vi "BUILD_uninstall core.vi"(6 "Buildlog":path, 8 "error in":errorcluster, 9 "args":string[](array[string]), 11 "appended path":path) -> (0 "error out":errorcluster)   [LabVIEW 2010]
uses:
  <vilib>/JKI/VIPM API/VIPM API_vipm_api.lvlib
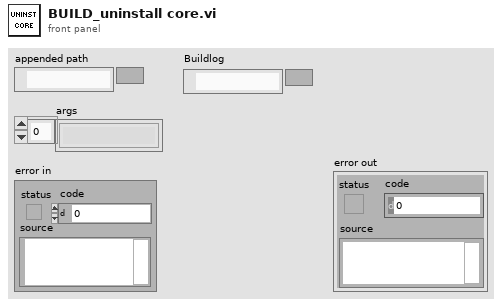
[diagram p1: front panel]
types:
  T1 = typedef "VIPM API_vipm_api.lvlib/Library Contents Cluster_vipm_api.ctl" = cluster{"Package Name":string, "Version":string, "Display Name":string, "Repository Name":string, "Company Name":string, "License Type":string, "Installed":bool, "Deprecated":bool, "Dependency or Conflict Problem":bool, "Downloaded":bool}
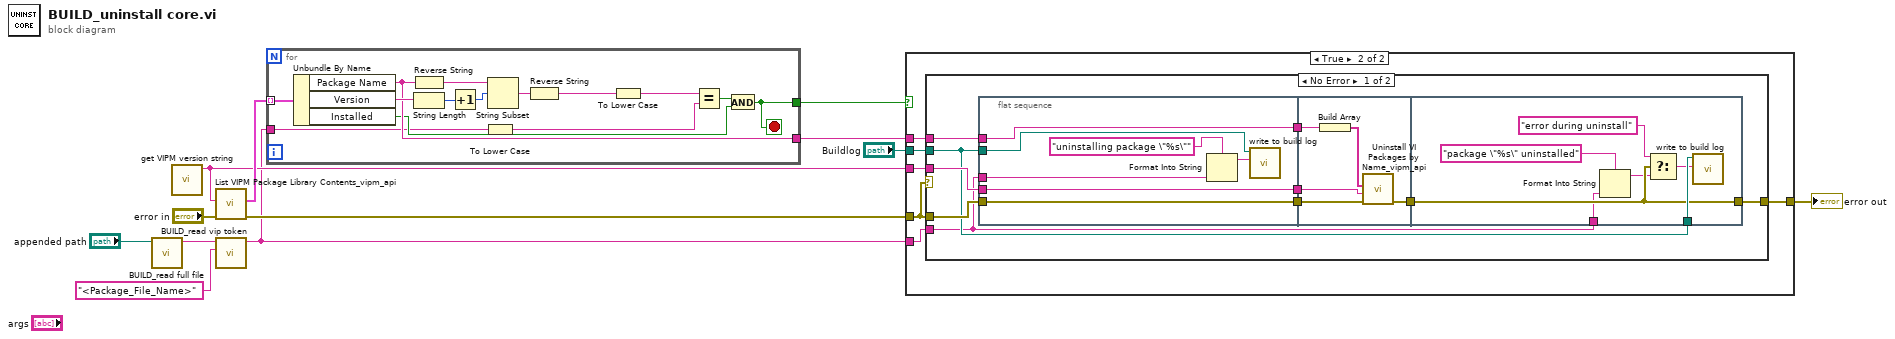
[diagram p0: block diagram]
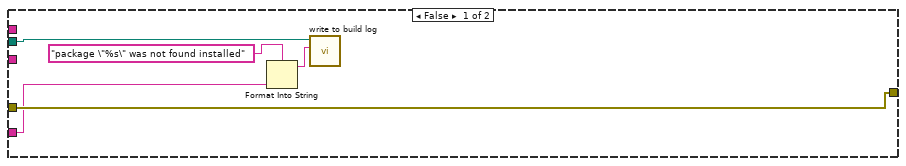
[diagram p2: hidden frame]
diagram:
  n1 = call "BUILD_read full file.vi"("vip file"="appended path") -> ("data"=w11:string)  [unwired: 9 in, 1 out]
  n2 = call "get VIPM version string.vi"() -> ("version string"=w3:string)  [unwired: 11 in]
  n3 = call <vilib>:"List VIPM Package Library Contents_vipm_api.vi"("error in (no error)"="error in", "LabVIEW Version"=w3) -> ("error out"=w7:errorcluster, "Library Contents []"=w6:T1[])  [unwired: 8 in]
  n4 = call "BUILD_read vip token.vi"("regular expression"="<Package_File_Name>", "data"=w11) -> ("trimmed string"=w1:string)  [unwired: 8 in, 1 out]
  n5 = for {
    tunnel: w6 -> [w26] mode=indexing
    tunnel: [w20] -> w8
    tunnel: [w16] -> w9
    tunnel: w1 -> [w15]
    stop <- w16 stop-if-true
    n6 = Unbundle By Name(w26) -> ("Package Name"=w20:string, "Version"=w25:string, "Installed"=w17:bool)
    n7 = Reverse String(1:w20) -> (0:w22:string)
    n8 = String Length(string=w25) -> (length=w24:i32)
    n9 = Increment(x=w24) -> (x+1=w23:i32)
    n10 = To Lower Case(string=w15) -> (all lower case string=w13:string)
    n11 = String Subset(string=w22, offset (0)=w23) -> (substring=w21:string)  [unwired: 1 in]
    n12 = Reverse String(1:w21) -> (0:w19:string)
    n13 = To Lower Case(string=w19) -> (all lower case string=w14:string)
    n14 = Equal?(x=w14, y=w13) -> (x = y?=w18:bool)
    n15 = And(x=w18, y=w17) -> (x .and. y?=w16:bool)
  }
  n16 = case shown="True" w9 {
    tunnel: [w31 w37] -> w5
    tunnel: w3 -> [_ w36]
    tunnel: w7 -> [w31 w34]
    tunnel: w8 -> [_ w35]
    tunnel: "Buildlog" -> [w30 w33]
    tunnel: w1 -> [w27 w32]
    frame False {
      n17 = Format Into String(format string="package \"%s\" was not found installed", w27) -> (resulting string=w29:string)  [unwired: 2 in, 1 out]
      n18 = call "write to build log.vi"("text"=w29, "log"=w30) -> ()  [unwired: 10 in]
    }
    frame True {
      n19 = case shown="No Error" w34 {
        tunnel: [w47 w67] -> w37
        tunnel: w36 -> [w46 _]
        tunnel: w34 -> [w45 w67]
        tunnel: w35 -> [w44 _]
        tunnel: w33 -> [w39 _]
        tunnel: w32 -> [w38 _]
        frame No Error {
          n20 = flat-sequence {
            tunnel: w44 -> [w52]
            tunnel: w45 -> [w53]
            tunnel: w46 -> [w54]
            tunnel: [w54] -> w43
            tunnel: [w53] -> w42
            tunnel: [w52] -> w41
            tunnel: w39 -> [w51]
            tunnel: w38 -> [w48]
            tunnel: w43 -> [w57]
            tunnel: w42 -> [w56]
            tunnel: w41 -> [w55]
            tunnel: [w58] -> w40
            tunnel: [w64] -> w47
            tunnel: w40 -> [w64]
            tunnel: w39 -> [w66]
            tunnel: w38 -> [w60]
            frame #0 {
              n21 = Format Into String(format string="uninstalling package \"%s\"", w48) -> (resulting string=w49:string)  [unwired: 2 in, 1 out]
              n22 = call "write to build log.vi"("text"=w49, "log"=w51) -> ()  [unwired: 10 in]
            }
            frame #1 {
              n23 = Build Array(w55) -> (w59:string[])
              n24 = call <vilib>:"Uninstall VI Packages by Name_vipm_api.vi"("error in (no error)"=w56, "LabVIEW Version"=w57, "Package Names to Uninstall []"=w59) -> ("error out"=w58:errorcluster)  [unwired: 8 in]
            }
            frame #2 {
              n25 = Format Into String(format string="package \"%s\" uninstalled", w60) -> (resulting string=w63:string)  [unwired: 2 in, 1 out]
              n26 = Select(t="error during uninstall", s=w64, f=w63) -> (s? t:f=w62:string)
              n27 = call "write to build log.vi"("text"=w62, "log"=w66) -> ()  [unwired: 10 in]
            }
          }
        }
        frame Error {
        }
      }
    }
  }
  "error out" <- w5
